vi "Тест_буфера_дублирвание_строк.vi"() -> ()   [LabVIEW 2013]
panel:
  out "x/y":dbl
  out "output array 2":dbl[](array[numeric])
  in  "Кол-во дубликатов окна":i32=5
  out "Подготовленный к отправке мажоритарный код":dbl[][](array[numeric])
  out "2-х массив на выходе 3":dbl[][](array[numeric])
  out "Кол-во строк массив":i32
  in  "Размер окна":i32=4
  out "Выход последовательного массива":dbl[](array[numeric])
  in  "Последовательный массив":i32=16
  out "Array":dbl[][](array[numeric])
  in  "Размер окна буффера":i32
  out "Количество бит":i32
  in  "Количество бит":i32=8
  out "Биты на выходе":dbl[](array[numeric])
  # "3"
  # "15"
  # "7"
  # "3"
  # "7"
  # "15"
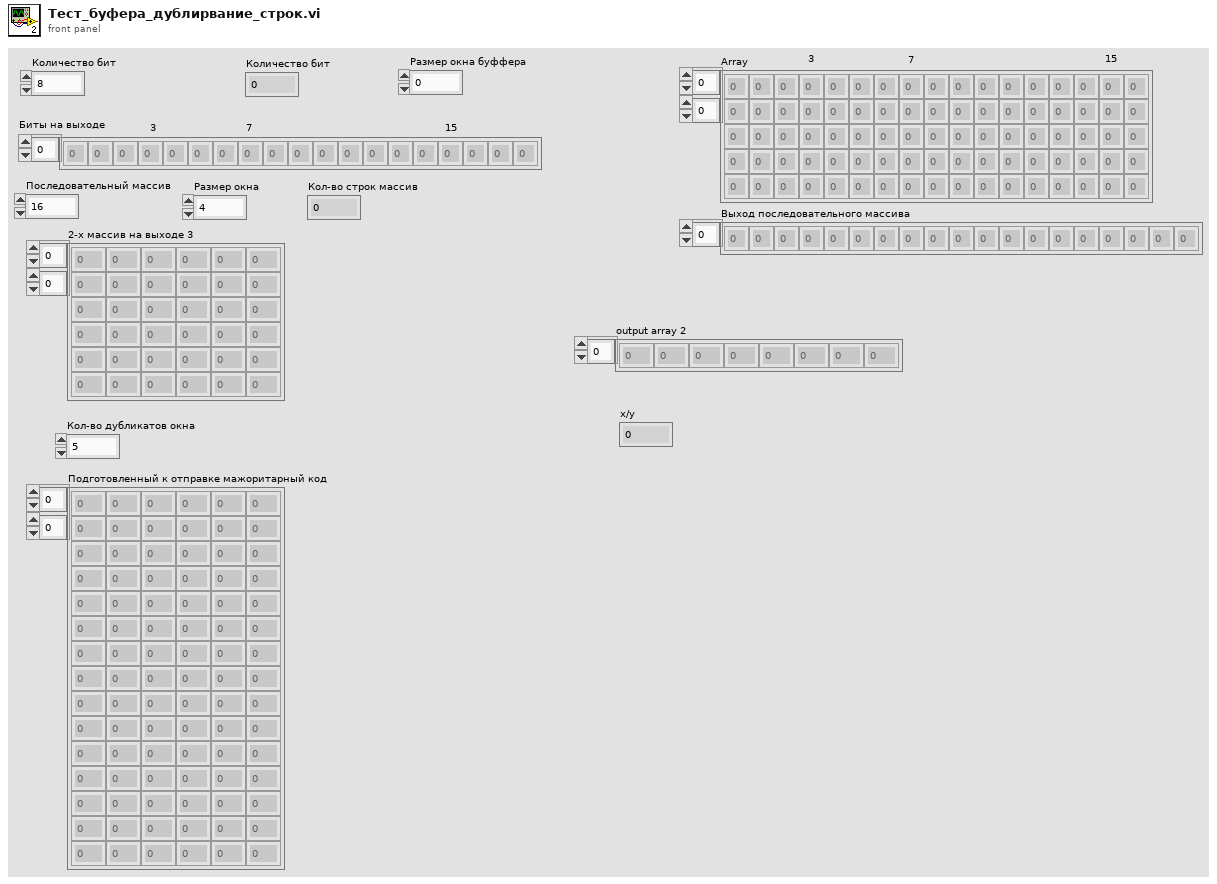
[diagram p1: front panel]
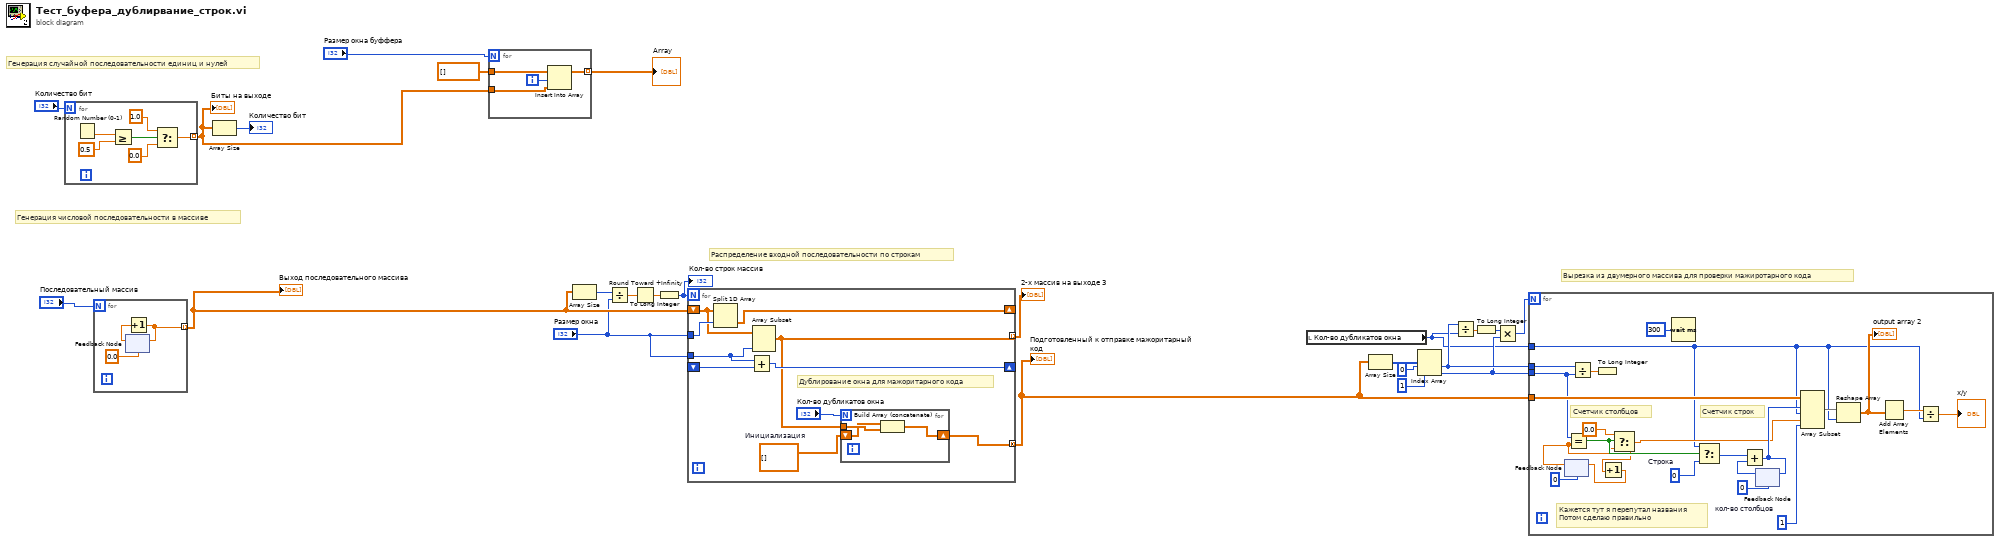
[diagram p0: block diagram]
diagram:
  # "Вырезка из двумерного массива для проверки мажиротарного кода"
  # "Распределение входной последовательности по строкам"
  # "Генерация числовой последовательности в массиве"
  # "Генерация случайной последовательности единиц и нулей"
  n1 = for {
    N: "Количество бит" -> [_]
    tunnel: [w25] -> w19 mode=indexing
    n2 = Random Number (0-1)() -> (number: 0 to 1=w30:dbl)
    n3 = Greater Or Equal?(x=w30, y=0.5) -> (x >= y?=w28:bool)
    n4 = Select(t=1.0, s=w28, f=0.0) -> (s? t:f=w25:dbl)
  }
  "Биты на выходе" <- w19
  n5 = for {
    N: "Последовательный массив" -> [_]
    tunnel: [w31] -> w16 mode=indexing
    n6 = feedback #1(0.0) -> (w33:dbl)
    n7 = Increment(x=w33) -> (x+1=w31:dbl)
    n8 = feedback-in #1(w31) -> ()
  }
  "Выход последовательного массива" <- w16
  n9 = Array Size(array=w19) -> (size(s)=→"Количество бит":i32)
  n10 = for {
    N: "Размер окна буффера" -> [_]
    tunnel: w19 -> [w35]
    tunnel: dbl[] [] -> [w36]
    tunnel: [w37] -> w22 mode=indexing
    i -> [w34]
    n11 = Insert Into Array(array=w36, index=w34, new element=w35) -> (w37:dbl[])
  }
  "Array" <- w22
  n12 = Array Size(array=w16) -> (size(s)=w17:i32)
  n13 = Divide(x=w17, y="Размер окна") -> (x/y=w15:dbl)
  n14 = Round Toward +Infinity(x=w15) -> (ceil(x): smallest int >= x=w14:dbl)
  n15 = To Long Integer(number=w14) -> (32bit integer=w11:i32)
  "Кол-во строк массив" <- w11
  n16 = for {
    N: w11 -> [_]
    shift-right: [w47] -> _
    shift-left: w16 -> [w45]
    tunnel: "Размер окна" -> [w46]
    shift-right: [w43] -> _
    shift-left: _ -> [w42]
    tunnel: "Размер окна" -> [w44]
    tunnel: [w40] -> w12 mode=indexing
    tunnel: [w39] -> w7 mode=concatenating
    w38 = dbl[][] []  # Инициализация
    # "Дублирование окна для мажоритарного кода"
    n17 = Split 1D Array(array=w45, index=w46) -> (second subarray=w47:dbl[])  [unwired: 1 out]
    n18 = Add(x=w44, y=w42) -> (x+y=w43:i32)
    n19 = Array Subset(array=w45, length=w44) -> (w40:dbl[])  [unwired: 1 in]
    n20 = for {
      N: "Кол-во дубликатов окна" -> [_]
      tunnel: w40 -> [w49]
      shift-right: [w50] -> w39
      shift-left: w38 -> [w48]
      n21 = Build Array (concatenate)(w48, w49) -> (w50:dbl[][])
    }
  }
  "2-х массив на выходе 3" <- w12
  "Подготовленный к отправке мажоритарный код" <- w7
  n22 = local read "Кол-во дубликатов окна"() -> (w1:i32)
  n23 = Array Size(array=w7) -> (size(s)=w10:i32[])
  n24 = Index Array(array=w10, index #1=0 ("index"), index #2=1 ("index")) -> (element #1=w6:i32, element #2=w5:i32)
  n25 = Divide(x=w6, y=w1) -> (x/y=w4:dbl)
  n26 = To Long Integer(number=w4) -> (32bit integer=w3:i32)
  n27 = Multiply(x=w3, y=w5) -> (x*y=w2:i32)
  n28 = for {
    N: w2 -> [_]
    tunnel: w7 -> [w71]
    tunnel: w5 -> [w61]
    tunnel: w6 -> [w69]
    tunnel: w1 -> [w52]
    w70 = 1  # кол-во столбцов
    w59 = 0  # Строка
    # "Кажется тут я перепутал названия  \nПотом сделаю правильно"
    # "Счетчик строк"
    # "Счетчик столбцов"
    n29 = feedback #2(0) -> (w57:dbl)
    n30 = Equal?(x=w61, y=w57) -> (x = y?=w63:bool)
    n31 = Divide(x=w69, y=w61) -> (x/y=w68:dbl)
    n32 = To Long Integer(number=w68) -> ()  [unwired: 1 out]
    n33 = Select(t=0.0, s=w63, f=w57) -> (s? t:f=w56:dbl)
    n34 = Increment(x=w56) -> (x+1=w55:dbl)
    n35 = feedback-in #2(w55) -> ()
    n36 = Wait (ms)(milliseconds to wait=u32 300) -> ()  [unwired: 1 out]
    n37 = Select(t=w52, s=w63, f=w59) -> (s? t:f=w60:i32)
    n38 = feedback #3(0) -> (w62:i32)
    n39 = Add(x=w60, y=w62) -> (x+y=w58:i32)
    n40 = feedback-in #3(w58) -> ()
    n41 = Array Subset(array=w71, index (row)=w58, length (row)=w52, index (col)=w56, length (col)=w70) -> (w72:dbl[][])
    n42 = Reshape Array(w72, w52) -> (w54:dbl[])
    "output array 2" <- w54
    n43 = Add Array Elements(numeric array=w54) -> (sum=w53:dbl)
    n44 = Divide(x=w53, y=w52) -> (x/y=→"x/y":dbl)
  }
